vi "Load Mice from PPL.vi"(11 "Mouse PPL":path) -> (0 "error out":errorcluster, 2 "Name":string, 3 "Mouse":refnum<class "Mouse.lvclass">)   [LabVIEW 2020, in "App.lvlib" / "MazeUI.lvclass"]
uses:
  MazeUI.lvclass
  build/ppl/maze.lvlibp/Mouse/Mouse.lvclass
  <vilib>/Utility/LVLibp/NI_PackedLibraryUtility.lvlib
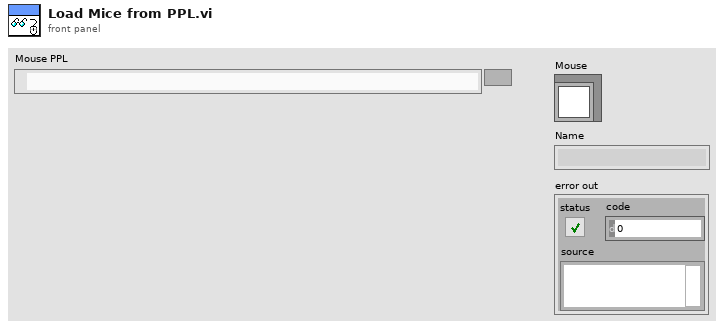
[diagram p1: front panel]
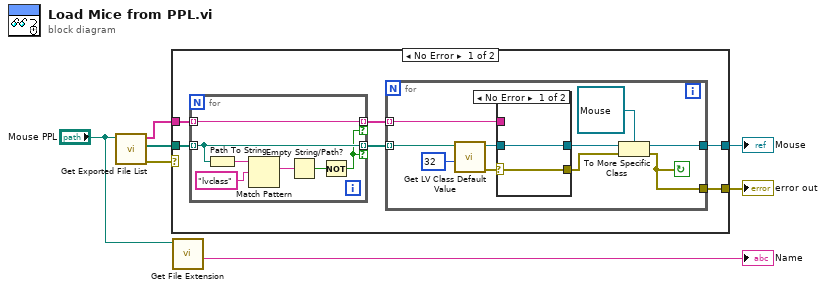
[diagram p0: block diagram]
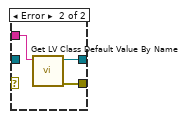
[diagram p2: hidden frame]
diagram:
  n1 = call <vilib>:"Get Exported File List.vi"("packed library path"="Mouse PPL") -> ("error out"=w4:errorcluster, "paths"=w5:path[], "qualified names"=w6:string[])  [unwired: 8 in]
  n2 = case shown="No Error" w4 {
    selector: w4 -> [_ w36]
    tunnel: [w9 _] -> w3
    tunnel: [w8 w36] -> w7
    tunnel: w6 -> [w12 _]
    tunnel: w5 -> [w10 _]
    frame No Error {
      n3 = for {
        tunnel: w10 -> [w31] mode=indexing
        tunnel: [w31] -> w13 mode=indexing if=w29
        tunnel: [w30] -> w11 mode=indexing if=w29
        tunnel: w12 -> [w30] mode=indexing
        n4 = Path To String(path=w31) -> (string=w35:string)
        n5 = Match Pattern(string=w35, regular expression="lvclass") -> (match substring=w33:string)  [unwired: 1 in, 3 out]
        n6 = Empty String/Path?(string/path=w33) -> (empty?=w32:bool)
        n7 = Not(x=w32) -> (.not. x?=w29:bool)
      }
      n8 = for {
        tunnel: w13 -> [w21] mode=indexing
        tunnel: [w22] -> w9
        tunnel: [w14] -> w8
        tunnel: w11 -> [w17] mode=indexing
        stop <- w14 continue-if-true
        n9 = call <vilib>:"Get LV Class Default Value.vi"("options"=u32 32, "class path"=w21) -> ("error out"=w19:errorcluster, "object"=w20:refnum<class>)  [unwired: 8 in]
        n10 = case shown="No Error" w19 {
          selector: w19 -> [w24 _]
          tunnel: w20 -> [w25 _]
          tunnel: [w25 w27] -> w18
          tunnel: w17 -> [_ w28]
          tunnel: [w24 w26] -> w16
          frame No Error {
          }
          frame Error {
            n11 = call <vilib>:"Get LV Class Default Value By Name.vi"("class name"=w28) -> ("error out"=w26:errorcluster, "object"=w27:refnum<class>)  [unwired: 9 in]
          }
        }
        n12 = To More Specific Class(target class=refnum<class "Mouse.lvclass"> refnum ("maze.lvlibp:Mouse.lvclass"), reference=w18, error in=w16) -> (specific class reference=w22:refnum<class "Mouse.lvclass">, error out=w14:errorcluster)
      }
    }
    frame Error {
    }
  }
  "error out" <- w7
  "Mouse" <- w3
  n13 = call <vilib>:"Get File Extension.vi"("file"="Mouse PPL") -> ("filename without extension"=→"Name":string)  [unwired: 6 in, 4 out]
